vi "Class Flag to Eum.vi"(8 "error in (no error)":errorcluster, 11 "Str":string) -> (0 "error out":errorcluster, 3 "Class":enum16{"Big", "Small"}(ring))   [LabVIEW 2014]
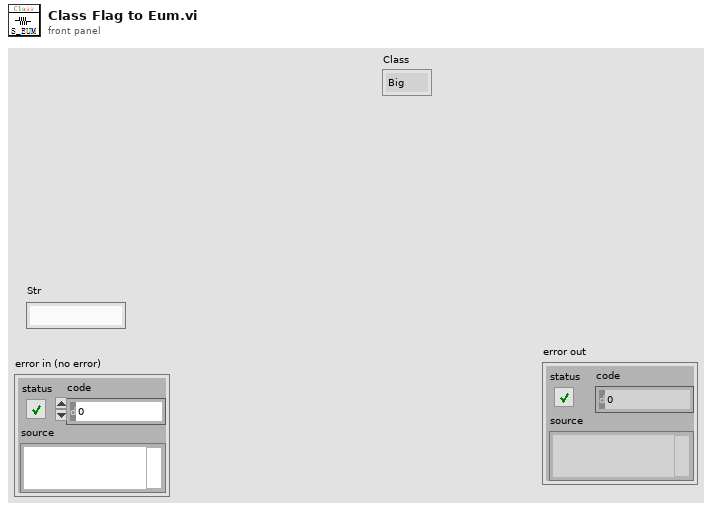
[diagram p1: front panel]
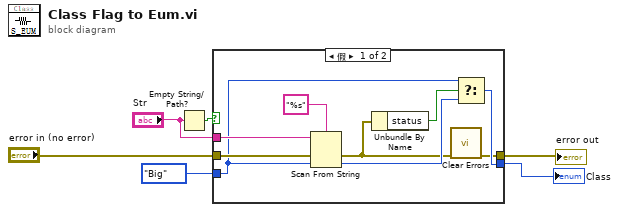
[diagram p0: block diagram]
diagram:
  n1 = Empty String/Path?(string/path="Str") -> (empty?=w6:bool)
  n2 = case shown="假" w6 {
    tunnel: [w9 w17] -> w2
    tunnel: "error in (no error)" -> [w15 w16]
    tunnel: "Str" -> [w14 _]
    tunnel: enum16{"Big", "Small"}."Big" ("Class") -> [w10 w17]
    tunnel: [w8 w16] -> w1
    frame False {
      n3 = Scan From String(format string="%s", input string=w14, error in=w15, default 1=w10) -> (error out=w7:errorcluster, output 1=w11:enum16{"Big", "Small"})  [unwired: 1 in, 2 out]
      n4 = Unbundle By Name(w7) -> ("status"=w12:bool)
      n5 = call <vilib>:"Clear Errors.vi"("error in (no error)"=w7) -> ("error out"=w8:errorcluster)  [unwired: 5 in, 1 out]
      n6 = Select(t=w10, s=w12, f=w11) -> (s? t:f=w9:enum16{"Big", "Small"})
    }
    frame True {
    }
  }
  "error out" <- w1
  "Class" <- w2
